vi "printgraph_V0.01.vi"(9 "reference 2":refnum<vi>, 10 "Fahrzeugdaten":refnum<vi>, 11 "XYGraph (Eingang)":refnum<vi>) -> ()   [LabVIEW 2014]
uses:
  <vilib>/Utility/NIReport.llb/NI_report.lvclass
  <vilib>/Utility/NIReport.llb/Append Report Text (str wrap).vi
panel:
  out "XY-Graph":cluster{dbl[], dbl[]}[](graph)
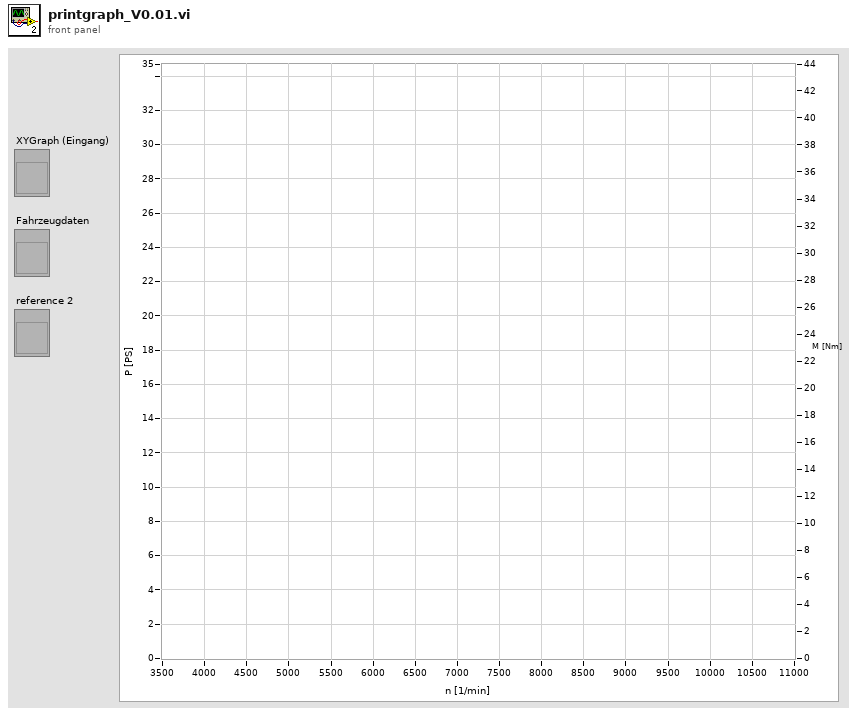
[diagram p1: front panel]
types:
  T1 = typedef "LVRangeTypeDef.ctl" = cluster{"Minimum":dbl, "Maximum":dbl, "Increment":dbl, "Minor Increment":dbl, "Start":dbl}
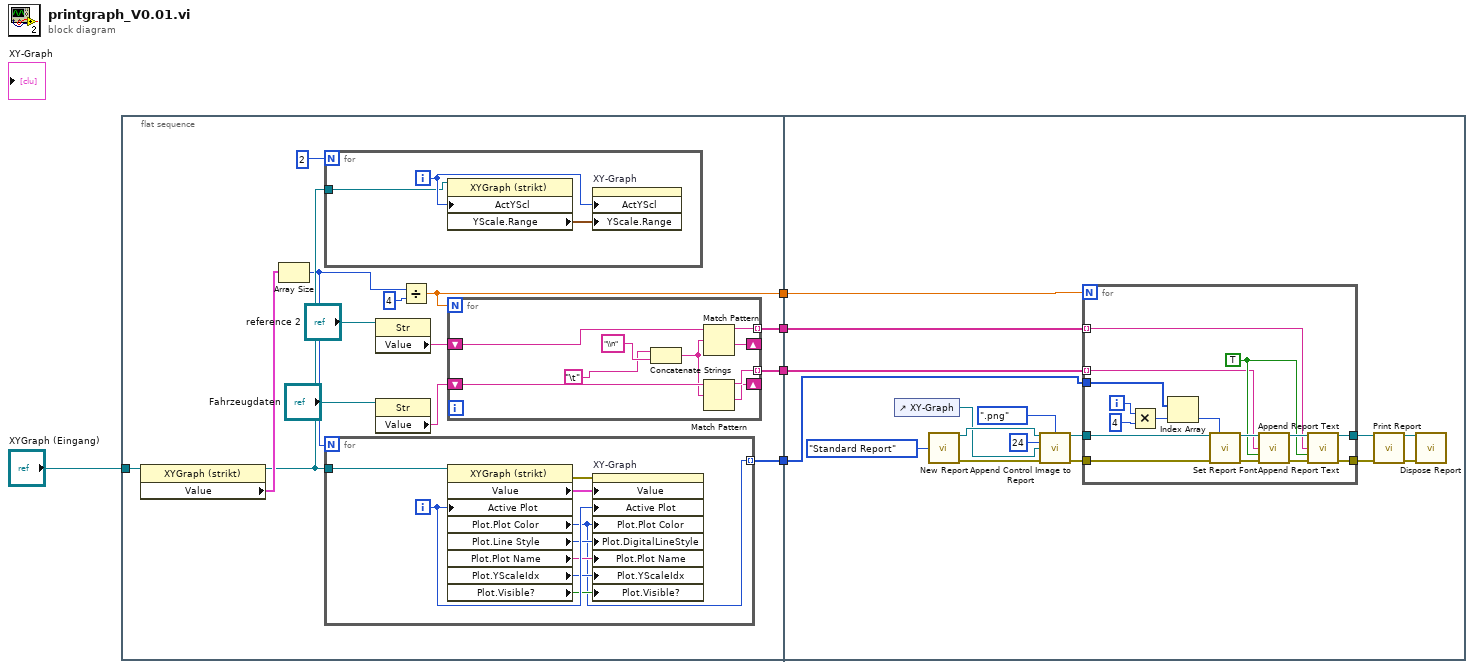
[diagram p0: block diagram]
diagram:
  n1 = flat-sequence {
    tunnel: "XYGraph (Eingang)" -> [w19]
    tunnel: [w13] -> w4
    tunnel: [w10] -> w3
    tunnel: [w9] -> w2
    tunnel: [w7] -> w1
    tunnel: w4 -> [w44]
    tunnel: w3 -> [w43]
    tunnel: w2 -> [w42]
    tunnel: w1 -> [w41]
    frame #0 {
      n2 = property on="Eigenschaftsknoten" class="XYGraph (strikt)"(reference=w19) -> (reference out=w16:refnum<vi>, "Value"=w18:cluster{dbl[], dbl[]}[])  [unwired: 1 in, 1 out]
      n3 = Array Size(array=w18) -> (size(s)=w6:i32)
      n4 = for {
        N: 2 -> [_]
        tunnel: w16 -> [w29]
        i -> [w30]
        n5 = property on="Eigenschaftsknoten" class="XYGraph (strikt)"(reference=w29, "ActYScl"=w30) -> ("YScale.Range"=w31:T1)  [unwired: 1 in, 2 out]
        n6 = property on="XY-Graph" class="XYGraph (strikt)"("ActYScl"=w30, "YScale.Range"=w31) -> ()  [unwired: 2 in, 2 out]
      }
      n7 = for {
        N: w6 -> [_]
        tunnel: w16 -> [w36]
        tunnel: [w32] -> w13 mode=indexing
        i -> [w40]
        n8 = property on="Eigenschaftsknoten" class="XYGraph (strikt)"(reference=w36, "Active Plot"=w40) -> (error out=w33:errorcluster, "Value"=w34:cluster{dbl[], dbl[]}[], "Plot.Plot Color"=w32:u32, "Plot.Line Style"=w39:u8, "Plot.Plot Name"=w38:string, "Plot.YScaleIdx"=w37:u32, "Plot.Visible?"=w35:bool)  [unwired: 1 in, 1 out]
        n9 = property on="XY-Graph" class="XYGraph (strikt)"(error in=w33, "Value"=w34, "Active Plot"=w40, "Plot.Plot Color"=w32, "Plot.DigitalLineStyle"=w39, "Plot.Plot Name"=w38, "Plot.YScaleIdx"=w37, "Plot.Visible?"=w35) -> ()  [unwired: 1 in, 2 out]
      }
      n10 = property class="Str"(reference="reference 2") -> ("Value"=w12:string)  [unwired: 1 in, 2 out]
      n11 = property class="Str"(reference="Fahrzeugdaten") -> ("Value"=w11:string)  [unwired: 1 in, 2 out]
      n12 = Divide(x=w6, y=u32 4) -> (x/y=w7:dbl)
      n13 = for {
        N: w7 -> [_]
        tunnel: [w25] -> w10 mode=indexing
        tunnel: [w26] -> w9 mode=indexing
        shift-right: [w22] -> _
        shift-left: w12 -> [w28]
        shift-right: [w21] -> _
        shift-left: w11 -> [w27]
        n14 = Concatenate Strings("\t", "\\n" ("Regulärer Ausdruck")) -> (w24:string)
        n15 = Match Pattern(string=w28, regular expression=w24) -> (before substring=w25:string, after substring=w22:string)  [unwired: 1 in, 2 out]
        n16 = Match Pattern(string=w27, regular expression=w24) -> (before substring=w26:string, after substring=w21:string)  [unwired: 1 in, 2 out]
      }
    }
    frame #1 {
      n17 = control-ref of="XY-Graph"() -> (w49:refnum<vi>)
      n18 = call <vilib>:"New Report.vi"("report type"=enum16{"Standard Report", "HTML"}."Standard Report") -> ("report out"=w56:refnum<class "NI_report.lvclass">, "error out"=w50:errorcluster)  [unwired: 13 in]
      n19 = call-dynamic "Append Control Image to Report.vi"("report in"=w56, "image file type (.jpg)"=enum16{".jpg", ".png"}.".png", "image depth"=24, "ctrl reference"=w49, "error in (no error)"=w50) -> ("report out"=w48:refnum<class "NI_report.lvclass">, "error out"=w47:errorcluster)  [unwired: 7 in, 2 out]
      n20 = for {
        N: w41 -> [_]
        tunnel: w47 -> [w70]
        tunnel: [w65] -> w45
        tunnel: w48 -> [w72]
        tunnel: [w66] -> w46
        tunnel: w44 -> [w63]
        tunnel: w43 -> [w58] mode=indexing
        tunnel: w42 -> [w57] mode=indexing
        i -> [w61]
        w64 = TRUE
        n21 = Multiply(x=w61, y=4) -> (x*y=w62:i32)
        n22 = Index Array(array=w63, index=w62) -> (element=w59:u32)
        n23 = call-dynamic "Set Report Font.vi"("report in"=w72, "text color (unchanged)"=w59, "error in (no error)"=w70) -> ("report out"=w71:refnum<class "NI_report.lvclass">, "error out"=w69:errorcluster)  [unwired: 10 in, 1 out]
        n24 = call-poly <vilib>:"Append Report Text.vi"("report in"=w71, "text"=w57, "append on new line? (F)"=w64, "error in (no error)"=w69) -> ("report out"=w68:refnum<class "NI_report.lvclass">, "error out"=w67:errorcluster)  [unwired: 8 in, 2 out]
        n25 = call-poly <vilib>:"Append Report Text.vi"("report in"=w68, "text"=w58, "append on new line? (F)"=w64, "error in (no error)"=w67) -> ("report out"=w66:refnum<class "NI_report.lvclass">, "error out"=w65:errorcluster)  [unwired: 8 in, 2 out]
      }
      n26 = call-dynamic "Print Report.vi"("report in"=w46, "error in (no error)"=w45) -> ("report out"=w54:refnum<class "NI_report.lvclass">, "error out"=w55:errorcluster)  [unwired: 12 in]
      n27 = call-dynamic "Dispose Report.vi"("report in"=w54, "error in (no error)"=w55) -> ()  [unwired: 13 in, 1 out]
    }
  }
